vi "Shift_006.vi"() -> ()   [LabVIEW 2019]
panel:
  in  "time threshold 2":dbl[unit]=5.0
  in  "Control Force 2":dbl[unit]=1000.0
  in  "time threshold 1":dbl[unit]=2.0
  in  "Control Force 1":dbl[unit]=1000.0
  in  "D":dbl[unit]=25.0
  out "Ep(tk)":dbl[unit][](array[numeric])
  out "Et(tk)":dbl[unit][](array[numeric])
  out "Ek(tk)":dbl[unit][](array[numeric])
  out "Et":cluster{dbl[unit][], dbl[unit][]}(graph)
  out "Ep":cluster{dbl[unit][], dbl[unit][]}(graph)
  out "Ek":cluster{dbl[unit][], dbl[unit][]}(graph)
  out "Et":dbl[unit][](graph)
  out "Ep":dbl[unit][](graph)
  out "Ek":dbl[unit][](graph)
  out "a":cluster{dbl[unit][], dbl[unit][]}(graph)
  out "v":cluster{dbl[unit][], dbl[unit][]}(graph)
  out "x":cluster{dbl[unit][], dbl[unit][]}(graph)
  out "time (tk)":dbl[unit][](array[numeric])
  out "a":dbl[unit][](graph)
  out "v":dbl[unit][](graph)
  out "x":dbl[unit][](graph)
  out "x(tk)":dbl[unit][](array[numeric])
  out "v(tk)":dbl[unit][](array[numeric])
  out "a(tk)":dbl[unit][](array[numeric])
  in  "M":dbl[unit]=100.0
  in  "k":dbl[unit]=1000.0
  in  "v0":dbl[unit]
  in  "x0":dbl[unit]=2.0
  in  "Dt":dbl[unit]=1e-05
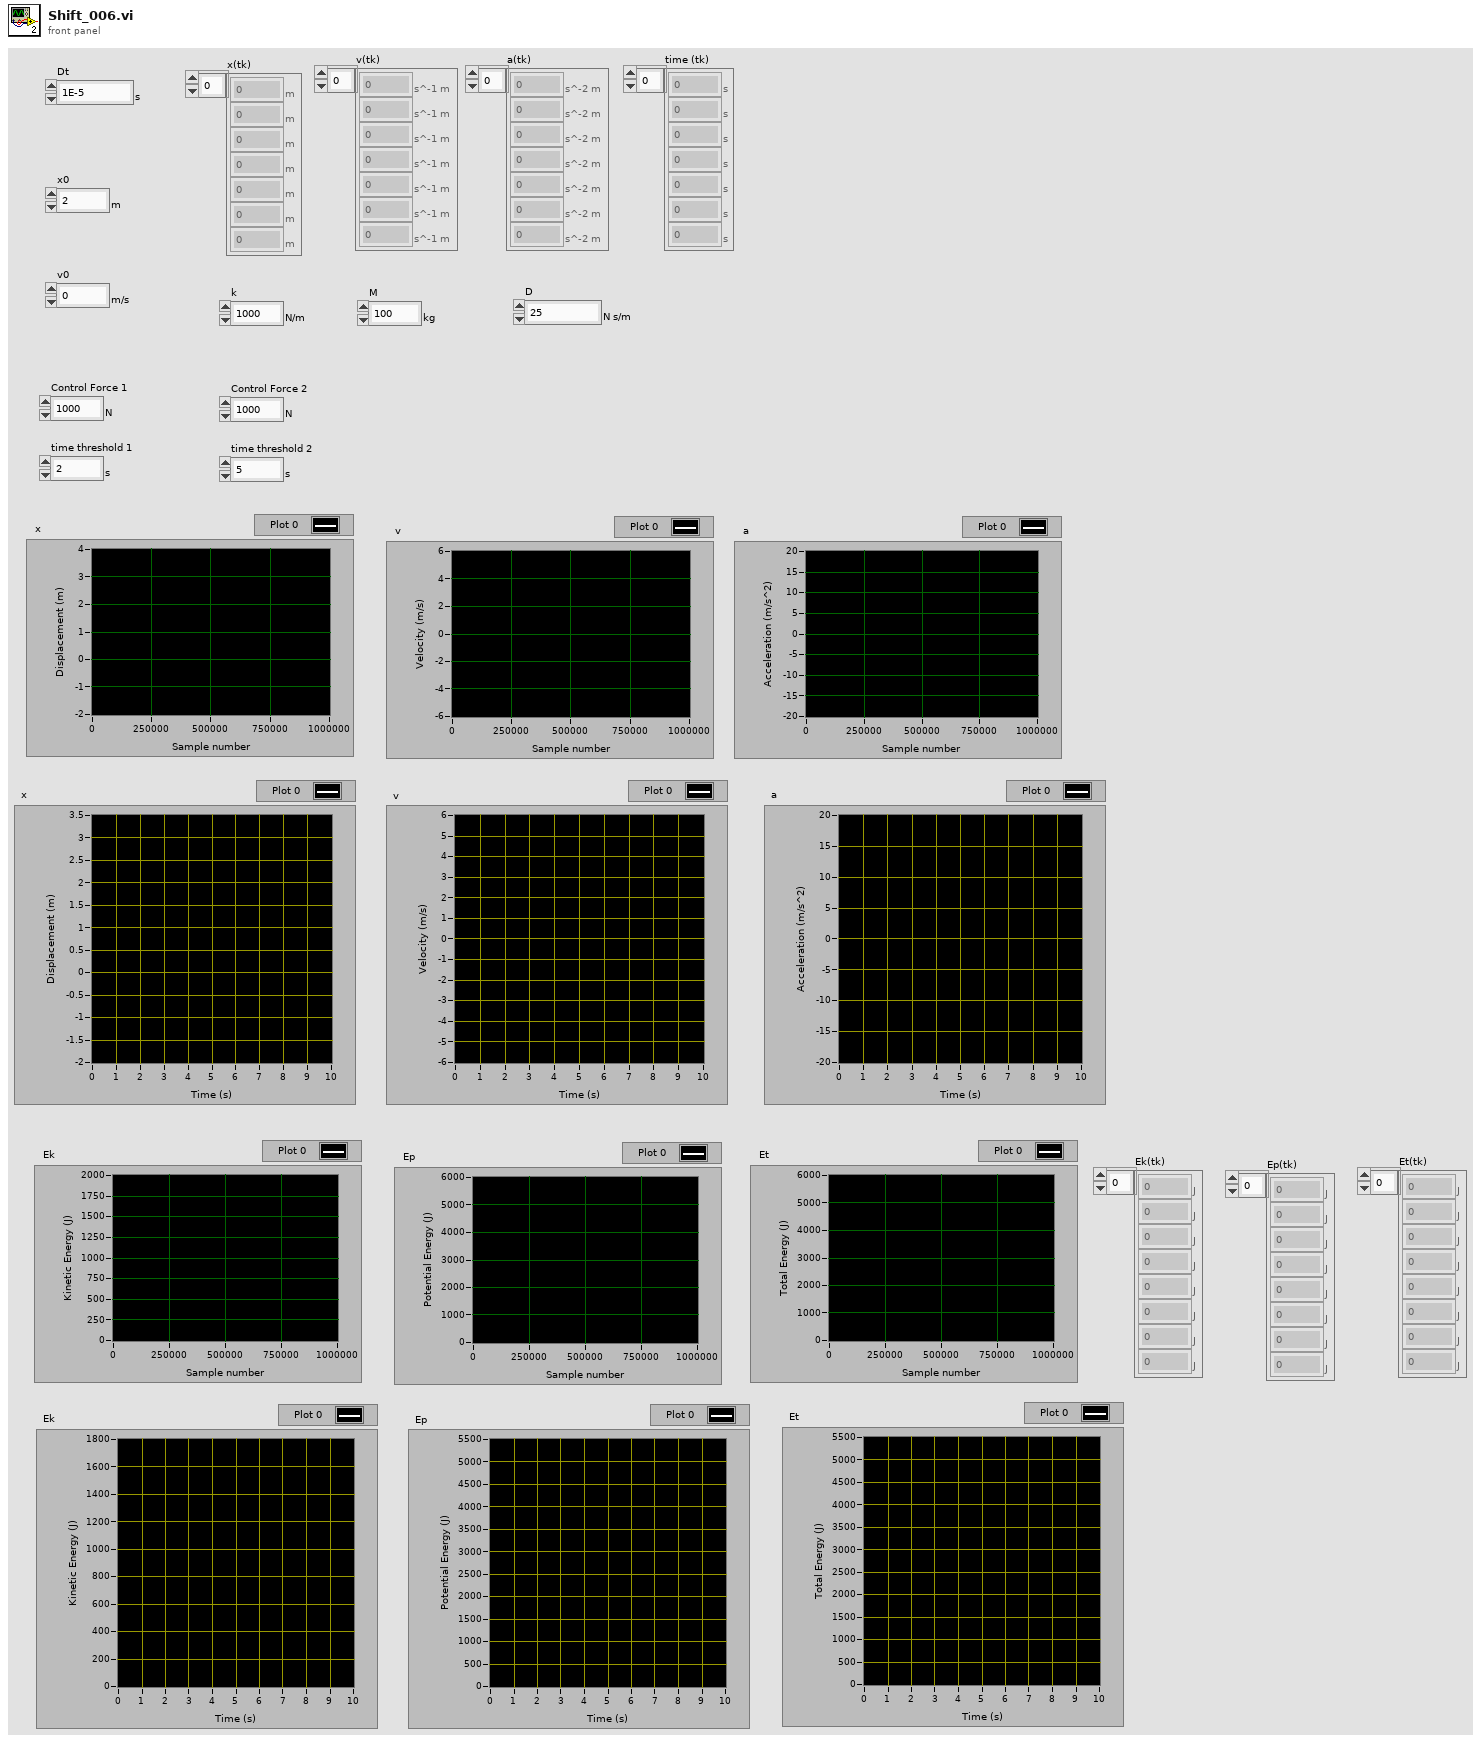
[diagram p1: front panel]
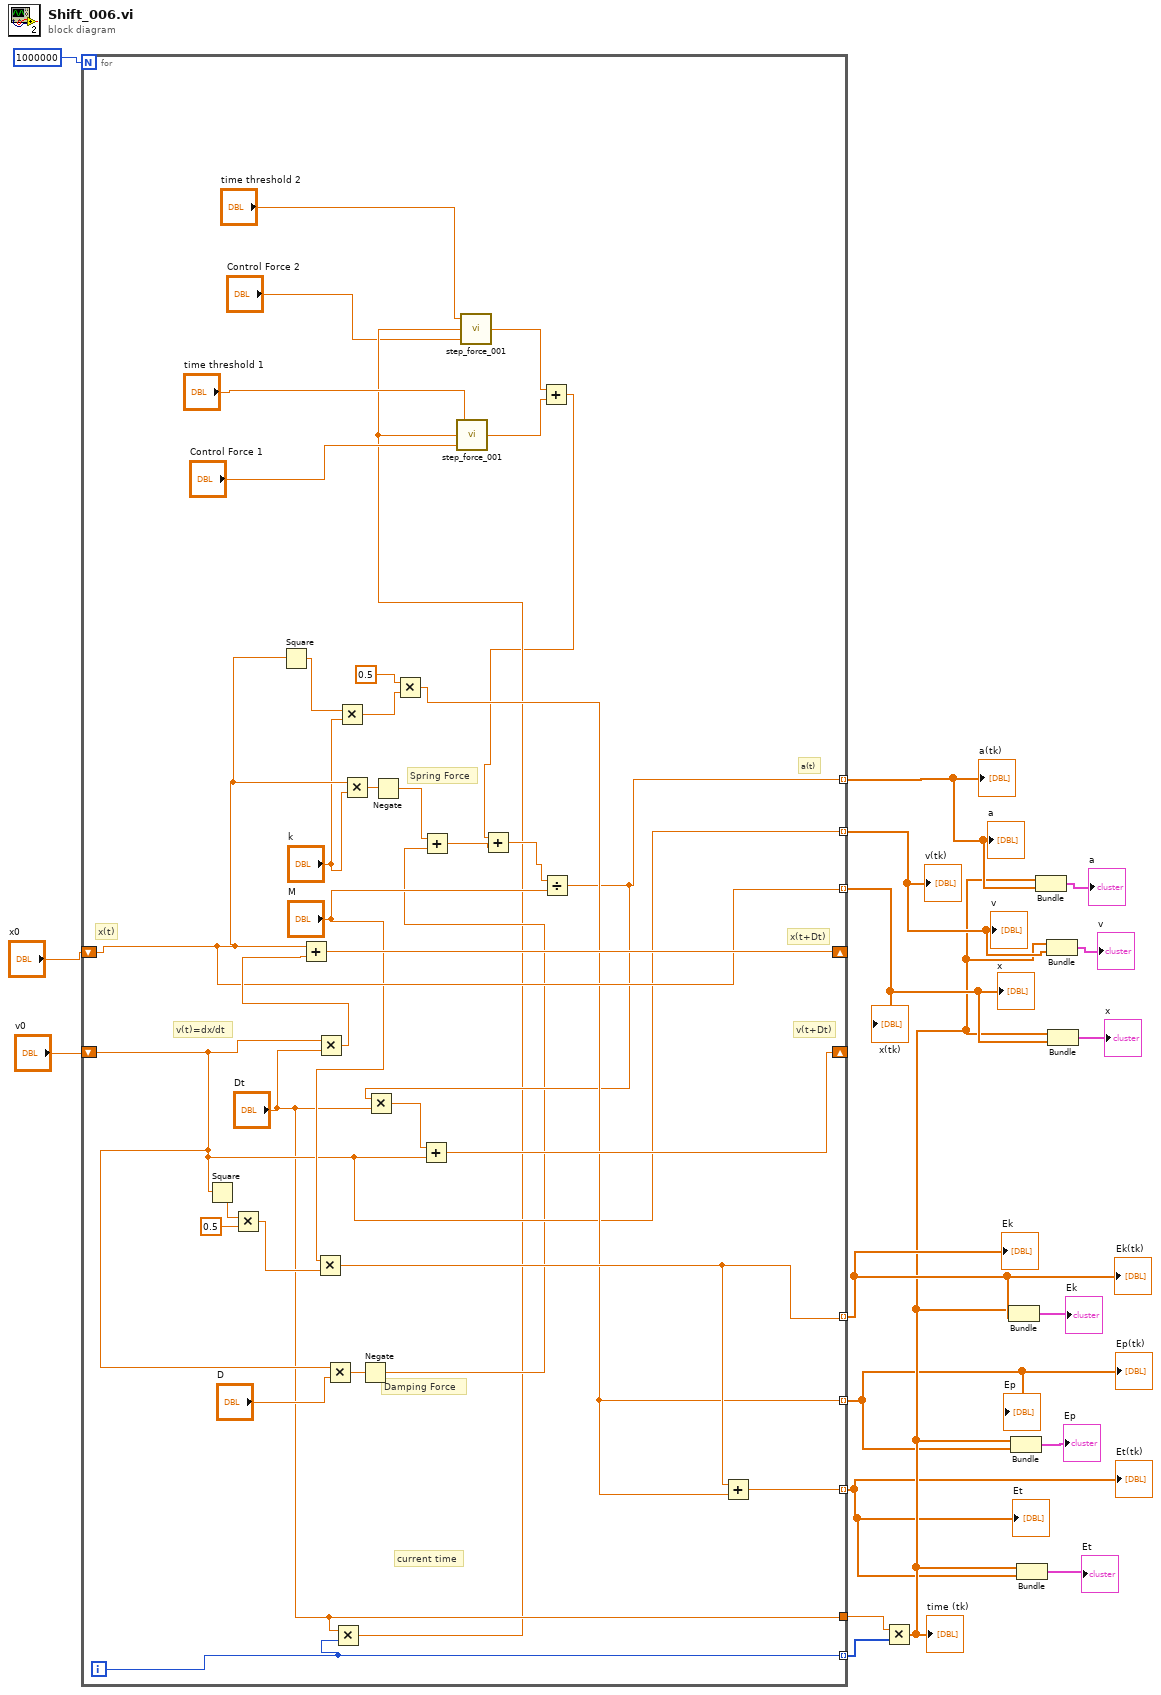
[diagram p0: block diagram]
diagram:
  n1 = for {
    N: 1000000 -> [_]
    shift-right: [w52] -> _
    shift-left: "x0" -> [w46]
    shift-right: [w49] -> _
    shift-left: "v0" -> [w36]
    tunnel: [w32] -> w10 mode=indexing
    tunnel: [w36] -> w9 mode=indexing
    tunnel: [w46] -> w8 mode=indexing
    tunnel: [w27] -> w14 mode=indexing
    tunnel: ["Dt"] -> w15
    tunnel: [w41] -> w4 mode=indexing
    tunnel: [w38] -> w1 mode=indexing
    tunnel: [w40] -> w2 mode=indexing
    i -> [w27]
    # "current time"
    # "Spring Force"
    # "Damping Force"
    # "a(t)"
    # "v(t+Dt)"
    # "x(t+Dt)"
    # "v(t)=dx/dt"
    # "x(t)"
    n2 = Square(x=w36) -> (x^2=w47:dbl[unit])
    n3 = Multiply(x=w47, y=0.5) -> (x*y=w42:dbl[unit])
    n4 = Square(x=w46) -> (x^2=w45:dbl[unit])
    n5 = Multiply(x="M", y=w42) -> (x*y=w41:dbl[unit])
    n6 = Multiply(x=w36, y="Dt") -> (x*y=w53:dbl[unit])
    n7 = Add(x=w46, y=w53) -> (x+y=w52:dbl[unit])
    n8 = Multiply(x=w36, y="D") -> (x*y=w35:dbl[unit])
    n9 = Multiply(x="Dt", y=w27) -> (x*y=w24:dbl[unit])
    n10 = Multiply(x=w45, y="k") -> (x*y=w44:dbl[unit])
    n11 = Multiply(x=w46, y="k") -> (x*y=w51:dbl[unit])
    n12 = Negate(x=w35) -> (-x=w31:dbl[unit])
    n13 = Negate(x=w51) -> (-x=w33:dbl[unit])
    n14 = Multiply(x=0.5, y=w44) -> (x*y=w38:dbl[unit])
    n15 = Add(x=w33, y=w31) -> (x+y=w30:dbl[unit])
    n16 = call "step_force_001.vi"("Control Force in"="Control Force 1", "Current time"=w24, "time threshold"="time threshold 1") -> ("Control Force out"=w21:dbl[unit])
    n17 = call "step_force_001.vi"("Control Force in"="Control Force 2", "Current time"=w24, "time threshold"="time threshold 2") -> ("Control Force out"=w20:dbl[unit])
    n18 = Add(x=w20, y=w21) -> (x+y=w19:dbl[unit])
    n19 = Add(x=w19, y=w30) -> (x+y=w29:dbl[unit])
    n20 = Divide(x=w29, y="M") -> (x/y=w32:dbl[unit])
    n21 = Multiply(x=w32, y="Dt") -> (x*y=w50:dbl[unit])
    n22 = Add(x=w50, y=w36) -> (x+y=w49:dbl[unit])
    n23 = Add(x=w41, y=w38) -> (x+y=w40:dbl[unit])
  }
  "a(tk)" <- w10
  "v(tk)" <- w9
  "x(tk)" <- w8
  "v" <- w9
  "a" <- w10
  "x" <- w8
  "Et" <- w2
  "Ek" <- w4
  "Ep" <- w1
  "Ek(tk)" <- w4
  "Et(tk)" <- w2
  "Ep(tk)" <- w1
  n24 = Multiply(x=w15, y=w14) -> (x*y=w3:dbl[unit][])
  "time (tk)" <- w3
  n25 = Bundle(w3, w4) -> (→"Ek":cluster{dbl[unit][], dbl[unit][]})  [unwired: 1 in]
  n26 = Bundle(w3, w1) -> (→"Ep":cluster{dbl[unit][], dbl[unit][]})  [unwired: 1 in]
  n27 = Bundle(w3, w2) -> (→"Et":cluster{dbl[unit][], dbl[unit][]})  [unwired: 1 in]
  n28 = Bundle(w3, w10) -> (→"a":cluster{dbl[unit][], dbl[unit][]})  [unwired: 1 in]
  n29 = Bundle(w3, w9) -> (→"v":cluster{dbl[unit][], dbl[unit][]})  [unwired: 1 in]
  n30 = Bundle(w3, w8) -> (→"x":cluster{dbl[unit][], dbl[unit][]})  [unwired: 1 in]
